vi "Numeric Control - Silver Dial.vi"() -> ()   [LabVIEW 2011]
doc: "Sample numeric display item."
uses:
  Silver Support LLB.llb/cluster_Screen Item Settings.ctl
  Silver Support LLB.llb/cluster_Graph Scale Settings.ctl
  Silver Support LLB.llb/cluster_Graph Plot Settings.ctl
  Silver Support LLB.llb/cluster_Graph Handler Message.ctl
  Silver Support LLB.llb/enum_Graph Handler Message.ctl
  Silver Support LLB.llb/sub_Display Template Handler Numeric.vi
  Silver Support LLB.llb/sub_Display Template Data Handler Numeric.vi
panel:
  in  "Meter Control":dbl(knob) scale=0.0..10.0
  in  "Item.Data":T1
  out "Label":string="Numeric"
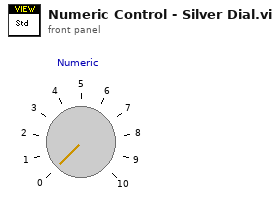
[diagram p1: front panel]
types:
  T1 = typedef "cluster_Screen Item Settings.ctl" = cluster{"Template VI":string, "Position X":i32, "Position Y":i32, "Custom":string, "Show Title Bar":bool, "ID":i32, "Always On Top":bool, "Allow Resize":bool, "Allow Minimize":bool, "Allow Close":bool, "Size to Screen":bool, "Screen.ID":i32, "State":enum16{"Normal", "New"}, "Title":string, "Window Bounds":cluster{"[0]":i16, "[1]":i16, "[2]":i16, "[3]":i16}, "Channel Ref":u64, "Unit":string, "Default Units?":bool, "Flash Limit?":bool, "Color 1":u32, "Color 2":u32, "Color 3":u32, "Color 4":u32, "Bck Color":u32, "Fore Color":u32, "Limit 1":dbl, "Limit 2":dbl, "Limit 3":dbl, "Limit 4":dbl, "Limit Mode 1":i32, "Limit Mode 2":i32, "Limit Mode 3":i32, "Limit Mode 4":i32, "Scale Precision":i32, "Scale Min":dbl, "Scale Max":dbl, "Format":i32, "Precision":i32, "Background Type":i32, "IDs":i32[], "Units":string[], "Labels":string[], "Scale Factor":dbl, "Scale Offset":dbl, "YScale Index":u32[], "XScale":T2, "YScales":T2[], "Plots":T3[], "Update Period":dbl, "History Length":dbl, "My.Ref":refnum<vi>, "Is Control?":bool, "Channel Paths":string[], "Custom Data":variant}
  T2 = typedef "cluster_Graph Scale Settings.ctl" = cluster{"Format":u8, "Precision":u8, "Fit":u8, "Label":string, "Use Default Label":bool, "Label Visible":bool, "Min":dbl, "Max":dbl}
  T3 = typedef "cluster_Graph Plot Settings.ctl" = cluster{"Bar Style":u8, "Fill To":i16, "Fill/PtColor":u32, "Line Style":u8, "Line Width":u8, "Color":u32, "Interp":u8, "Point Style":u8}
  T4 = typedef "cluster_Graph Handler Message.ctl" = cluster{"Message":T5, "Data":variant}
  T5 = typedef "enum_Graph Handler Message.ctl" = enum16{"None", "Stop", "Hold", "Update Channels", "New Settings", "Control Value", "Edit Value"}
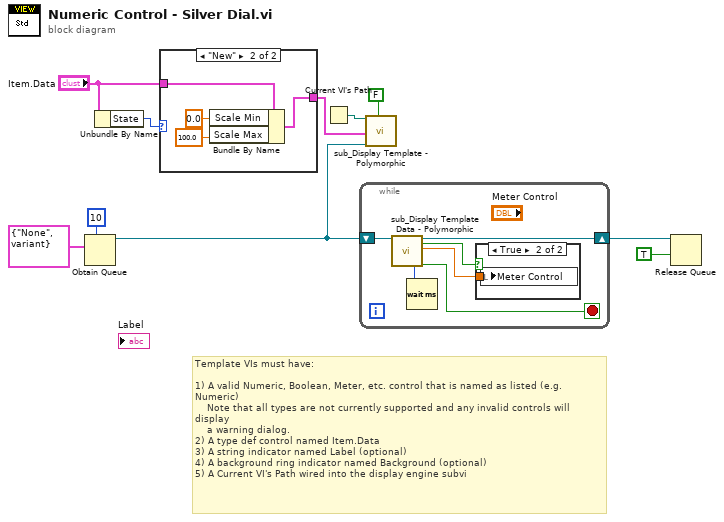
[diagram p0: block diagram]
diagram:
  # "Template VIs must have:\n\n1) A valid Numeric, Boolean, Meter, etc. control that is named as listed (e.g. Numeric)\n    Note that all types are not currently supported and any invalid controls will display\n    a warning dialog.\n2) A type def control named Item.Data\n3) A string indicator named Label (optional)\n4) A background ring indicator named Background (optional)\n5) A Current VI's Path wired into the display engine subvi"
  n1 = Obtain Queue(max queue size (-1, unlimited)=10, element data type=T4 {"Message"=enum."None", "Data"=variant} ("Message")) -> (queue out=w5:refnum<queue>)  [unwired: 2 in, 3 out]
  n2 = Unbundle By Name("Item.Data") -> ("State"=w2:enum16{"Normal", "New"})
  n3 = case shown="\"New\"" w2 {
    tunnel: [w11 w15] -> w1
    tunnel: "Item.Data" -> [w11 w12]
    frame Default {
    }
    frame "New" {
      n4 = Bundle By Name(cluster=w12, "Scale Min"=0.0, "Scale Max"=100.0) -> (w15:T1)
    }
  }
  n5 = Current VI's Path() -> (path=w10:path)
  n6 = while {
    shift-right: [w21] -> w9
    shift-left: w5 -> [w20]
    stop <- w18 stop-if-true
    n7 = call-poly "sub_Display Template Data - Polymorphic.vi"("queue"=w20) -> ("Wait.Time"=w19:u32, "queue out"=w21:refnum<queue>, "Update.Value"=w16:bool, "Numeric.Value"=w17:dbl, "Stop"=w18:bool)  [unwired: 14 out]
    n8 = Wait (ms)(milliseconds to wait=w19) -> ()  [unwired: 1 out]
    n9 = case shown="True" w16 {
      tunnel: w17 -> [_ w22]
      frame False {
      }
      frame True {
        n10 = local write "Meter Control"(w22) -> ()
      }
    }
  }
  n11 = call-poly "sub_Display Template - Polymorphic.vi"("Parent.Path"=w10, "Item.Data"=w1, "queue"=w5, "Use Transparency?"=FALSE) -> ()  [unwired: 16 out]
  n12 = Release Queue(queue=w9, force destroy? (F)=TRUE) -> ()  [unwired: 1 in, 3 out]
